vi "Driver Arrays.vi"(8 "error in":errorcluster, 9 "Value":i32, 10 "Index":i32, 11 "Curr Operation":T1(ring)) -> (0 "error out":errorcluster, 1 "Outport arr":i32[](array[numeric]), 2 "Value":i32, 3 "Inport arr":i32[](array[numeric]))   [LabVIEW 2025, in "Runtime Configuration Support Inline Async Example Engine.lvlib"]
uses:
  Runtime Configuration Support Inline Async Example Engine.lvlib
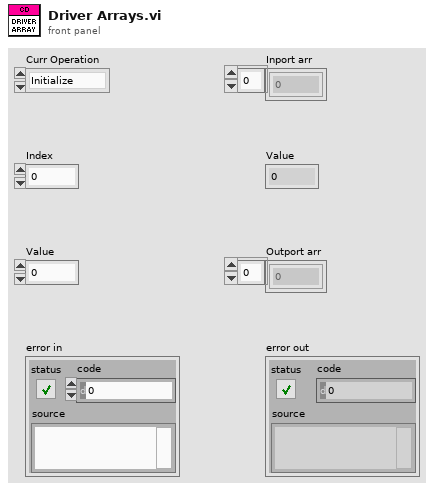
[diagram p1: front panel]
types:
  T1 = enum16{"Initialize", "Set In Val", "Get In Val", "Set Block", "Set Out Val", "Get Out Val", "Get In Array", "Get Out Array"}
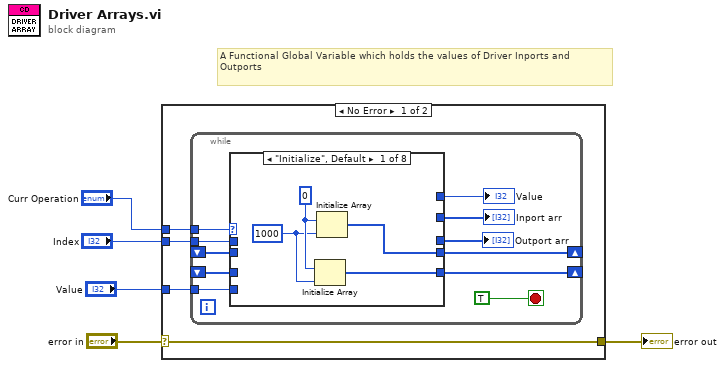
[diagram p0: block diagram]
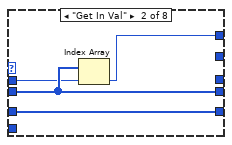
[diagram p2: hidden frame]
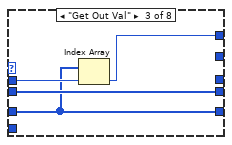
[diagram p3: hidden frame]
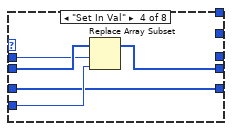
[diagram p4: hidden frame]
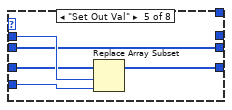
[diagram p5: hidden frame]
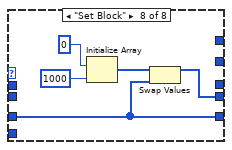
[diagram p8: hidden frame]
diagram:
  # "A Functional Global Variable which holds the values of Driver Inports and Outports"
  n1 = case shown="No Error" "error in" {
    selector: "error in" -> [w9 w52]
    tunnel: [w9 w52] -> w4
    tunnel: "Curr Operation" -> [w8 _]
    tunnel: "Index" -> [w7 _]
    tunnel: "Value" -> [w6 _]
    frame No Error {
      n2 = while {
        shift-right: [w15] -> _
        shift-left: _ -> [w18]
        tunnel: w8 -> [w19]
        tunnel: w7 -> [w17]
        tunnel: w6 -> [w16]
        shift-right: [w12] -> _
        shift-left: _ -> [w13]
        stop <- TRUE stop-if-true
        n3 = case shown="\"Initialize\", Default" w19 {
          tunnel: w18 -> [_ w28 w32 w37 w38 w43 w46 _]
          tunnel: [w24 w28 w32 w34 w38 w43 w46 w47] -> w15
          tunnel: w17 -> [_ w27 w31 w36 w42 _ _ _]
          tunnel: w16 -> [_ _ _ w35 w41 _ _ _]
          tunnel: [_ w26 w30 _ _ _ _ _] -> w14
          tunnel: w13 -> [_ w25 w29 w33 w40 w44 w45 w48]
          tunnel: [w21 w25 w29 w33 w39 w44 w45 w48] -> w12
          tunnel: [_ _ _ _ _ w43 _ _] -> w11
          tunnel: [_ _ _ _ _ _ w45 _] -> w10
          frame "Initialize", Default {
            w22 = 1000 ("dimension size")
            w23 = 0 ("element")
            n4 = Initialize Array(w23, w22) -> (w21:i32[])
            n5 = Initialize Array(w23, w22) -> (w24:i32[])
          }
          frame "Get In Val" {
            n6 = Index Array(array=w28, index=w27) -> (element=w26:i32)
          }
          frame "Get Out Val" {
            n7 = Index Array(array=w29, index=w31) -> (element=w30:i32)
          }
          frame "Set In Val" {
            n8 = Replace Array Subset(array=w37, new element=w35, index=w36) -> (w34:i32[])
          }
          frame "Set Out Val" {
            n9 = Replace Array Subset(array=w40, new element=w41, index=w42) -> (w39:i32[])
          }
          frame "Get In Array" {
          }
          frame "Get Out Array" {
          }
          frame "Set Block" {
            n10 = Initialize Array(0 ("element"), 1000 ("dimension size")) -> (w49:i32[])
            n11 = Swap Values(12:w49, 14:w48) -> (1:w47:i32[])  [unwired: 1 in, 1 out]
          }
        }
        "Inport arr" <- w11
        "Value" <- w14
        "Outport arr" <- w10
      }
    }
    frame Error {
    }
  }
  "error out" <- w4
